vi "TimerAssert.vi"(0 "error in (no error)":errorcluster, 1 "Label":string, 2 "Assert Only? (F)":bool, 5 "Expected Time":ext, 7 "Tolerance":ext=0.00000100000000000000000004, 11 "Start Time in":dbl, 14 "Use Percentage of X (F)":bool) -> (4 "error out":errorcluster, 15 "Start Time out":dbl)   [LabVIEW 2016, in "AssertTimer.lvlib"]
uses:
  AssertTimer.lvlib
  <vilib>/addons/_JKI Toolkits/Caraya/classes/Assert/Assert Almost Equal_Float.vi
  <vilib>/addons/_JKI Toolkits/Caraya/classes/Assert/Assert Equal Value_Variant.vi
  <vilib>/addons/_JKI Toolkits/Caraya/classes/Assert/Assert.lvclass
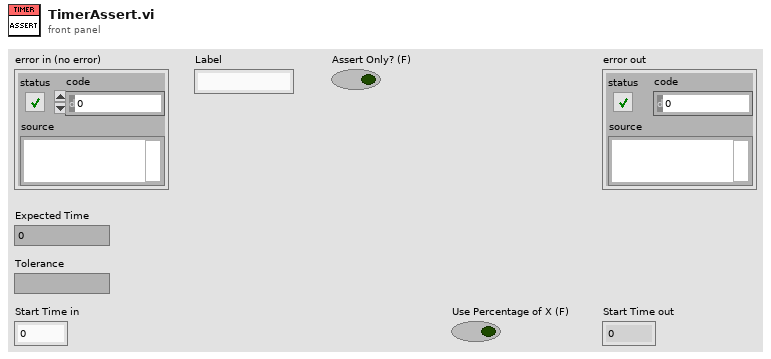
[diagram p1: front panel]
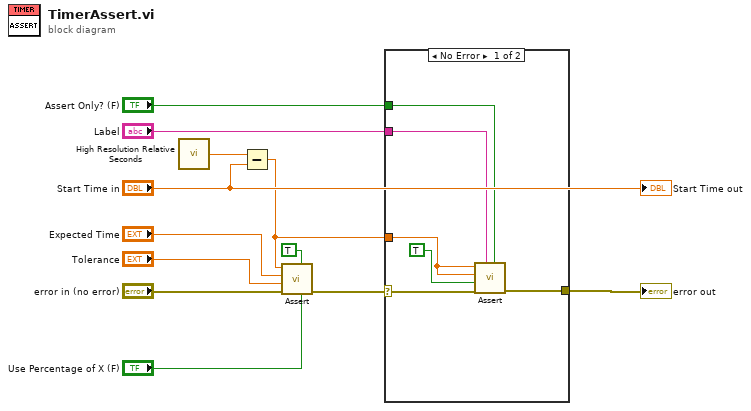
[diagram p0: block diagram]
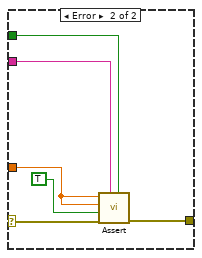
[diagram p2: hidden frame]
diagram:
  n1 = call <vilib>:"High Resolution Relative Seconds.vi"() -> ("relative seconds"=w8:dbl)
  n2 = Subtract(x=w8, y="Start Time in") -> (x-y=w4:dbl)
  n3 = call-poly <vilib>:"Assert.vi"("Use Percentage of X (F)"="Use Percentage of X (F)", "Assert Only? (F)"=TRUE, "error in (no error)"="error in (no error)", "Tolerance"="Tolerance", "Y"="Expected Time", "X"=w4) -> ("error out"=w6:errorcluster)  [unwired: 5 in]
  n4 = case shown="No Error" w6 {
    selector: w6 -> [w14 w22]
    tunnel: "Label" -> [w18 w24]
    tunnel: w4 -> [w16 w20]
    tunnel: "Assert Only? (F)" -> [w17 w23]
    tunnel: [w13 w21] -> w5
    frame No Error {
      n5 = call-poly <vilib>:"Assert.vi"("Assert Only? (F)"=w17, "Label"=w18, "error in (no error)"=w14, "Register with caller test (F)"=TRUE, "Y"=w16, "X"=w16) -> ("error out"=w13:errorcluster)  [unwired: 5 in]
    }
    frame Error {
      n6 = call-poly <vilib>:"Assert.vi"("Assert Only? (F)"=w23, "Label"=w24, "error in (no error)"=w22, "Register with caller test (F)"=TRUE, "Y"=w20, "X"=w20) -> ("error out"=w21:errorcluster)  [unwired: 5 in]
    }
  }
  "error out" <- w5
  "Start Time out" <- "Start Time in"
